vi "square-wave-generator.vi"(1 "Slope":dbl=1.0 format="%.2f", 3 "Width":dbl=140.0 format="%.2f", 4 "Height":dbl=120.0 format="%.2f", 5 "Period":dbl=310.0 format="%.2f", 6 "Length":i32=1000) -> (0 "Waveform Graph":dbl[](graph))   [LabVIEW 2017]
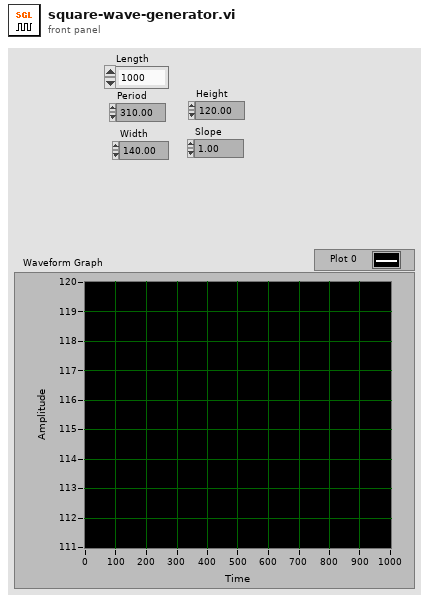
[diagram p1: front panel]
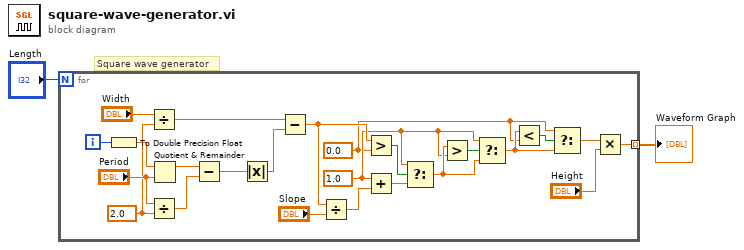
[diagram p0: block diagram]
diagram:
  # "Square wave generator"
  n1 = for {
    N: "Length" -> [_]
    tunnel: [w7] -> w1 mode=indexing
    i -> [w26]
    w3 = 0.0 ("t")
    w4 = 1.0 ("t")
    w5 = 2.0 ("y")
    n2 = To Double Precision Float(number=w26) -> (double precision float=w6:dbl)
    n3 = Divide(x="Width", y=w5) -> (x/y=w16:dbl)
    n4 = Divide(x="Period", y=w5) -> (x/y=w20:dbl)
    n5 = Quotient & Remainder(x=w6, y="Period") -> (x-y*floor(x/y)=w21:dbl)  [unwired: 1 out]
    n6 = Subtract(x=w21, y=w20) -> (x-y=w19:dbl)
    n7 = Absolute Value(x=w19) -> (abs(x)=w17:dbl)
    n8 = Subtract(x=w16, y=w17) -> (x-y=w13:dbl)
    n9 = Divide(x=w13, y="Slope") -> (x/y=w12:dbl)
    n10 = Greater?(x=w13, y=w3) -> (0:w15:bool)
    n11 = Add(x=w4, y=w12) -> (x+y=w11:dbl)
    n12 = Select(t=w4, s=w15, f=w11) -> (s? t:f=w10:dbl)
    n13 = Greater?(x=w10, y=w4) -> (0:w24:bool)
    n14 = Select(t=w4, s=w24, f=w10) -> (s? t:f=w22:dbl)
    n15 = Less?(x=w22, y=w3) -> (x < y?=w23:bool)
    n16 = Select(t=w3, s=w23, f=w22) -> (s? t:f=w8:dbl)
    n17 = Multiply(x=w8, y="Height") -> (x*y=w7:dbl)
  }
  "Waveform Graph" <- w1
